vi "readRange.vi"(8 "error in (no error)":errorcluster, 10 "range":string, 11 "FileReader in":refnum<class "FileReader.lvclass">) -> (0 "error out":errorcluster, 2 "range":dbl[](array[numeric]), 3 "FileReader out":refnum<class "FileReader.lvclass">)   [LabVIEW 2011, in "Tools.lvlib" / "Filing.lvlib" / "FileReader.lvclass"]
uses:
  FileReader.lvclass
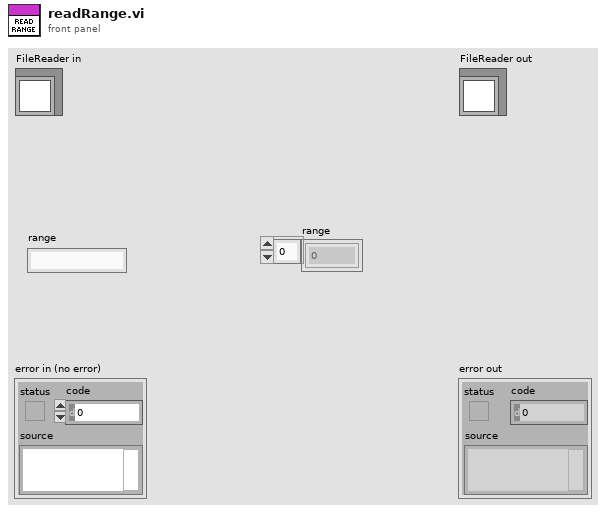
[diagram p1: front panel]
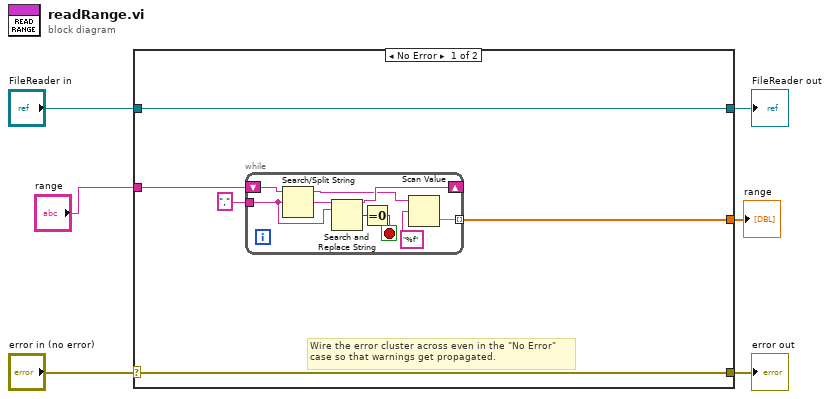
[diagram p0: block diagram]
diagram:
  n1 = case shown="No Error" "error in (no error)" {
    selector: "error in (no error)" -> [w10 w22]
    tunnel: [w10 w22] -> w5
    tunnel: [w11 w21] -> w3
    tunnel: "FileReader in" -> [w11 w21]
    tunnel: "range" -> [w8 _]
    tunnel: [w7 _] -> w1
    frame No Error {
      # "Wire the error cluster across even in the \"No Error\"\ncase so that warnings get propagated."
      n2 = while {
        tunnel: "," ("search string/char (-)") -> [w18]
        tunnel: [w14] -> w7 mode=indexing
        shift-right: [w13] -> _
        shift-left: w8 -> [w20]
        stop <- w16 stop-if-true
        n3 = Search/Split String(string=w20, search string/char (-)=w18) -> (substring before match=w12:string, match + rest of string=w19:string)  [unwired: 1 in, 1 out]
        n4 = Search and Replace String(input string=w19, search string=w18) -> (result string=w13:string, number of replacements=w17:i32)  [unwired: 6 in, 2 out]
        n5 = Equal To 0?(x=w17) -> (x = 0?=w16:bool)
        n6 = Scan Value(string=w12, format string="%f") -> (value=w14:dbl)  [unwired: 1 in, 1 out]
      }
    }
    frame Error {
    }
  }
  "error out" <- w5
  "FileReader out" <- w3
  "range" <- w1
